vi "3G-PHY-Layer-Complete-System.vi"() -> ()   [LabVIEW 2017]
uses:
  <vilib>/addons/Modulation/Digital/Channel Coding/MT Convolutional Encoder (Rate).vi
  <vilib>/addons/Modulation/Analog/support/mod_Set Error Source.vi
  <vilib>/addons/Modulation/Digital/Support/Common/Validators/mod_Validate Bit Stream.vi
  <vilib>/addons/Modulation/Digital/Channel Coding/Convolutional codes/mod_Convolutional encoder.vi
  <vilib>/addons/Modulation/Digital/Support/Common/Validators/mod_AWGN Validate.vi
  <vilib>/addons/Modulation/Digital/Impairments/subVIs/mod_createSeeds.vi
  <vilib>/addons/Modulation/Digital/Channel Coding/Convolutional codes/subVIs/mod_Generate encoder tap connections.vi
  <vilib>/addons/Modulation/Digital/Channel Coding/Convolutional codes/subVIs/mod_Perform convolutional encoding.vi
  <vilib>/addons/Modulation/Digital/Channel Coding/Block codes/subVIs/mod_Buffer block code info (I8).vi
  <vilib>/addons/Modulation/Digital/Channel Coding/Convolutional codes/subVIs/mod_Generate valid reset (convolutional, I8).vi
  <vilib>/addons/Modulation/Digital/Support/Common/Validators/mod_Validate Samples Per Symbol.vi
  <vilib>/addons/Modulation/Analog/support/Validators/mod_Validate Complex Waveform.vi
  <vilib>/addons/Modulation/Analog/support/Validators/mod_WFErrorHandler.vi
  <vilib>/addons/Modulation/Digital/General/MT Generate Bits (Fibonacci, PN Order).vi
  <vilib>/addons/Modulation/Digital/Support/Common/Validators/mod_Generate Filter Coefficients Validate.vi
  <vilib>/addons/Modulation/Digital/General/subVIs/mod_Generate Filter Coefficients.vi
  <vilib>/addons/Modulation/Digital/General/MT Generate PSK System Parameters(M).vi
  <vilib>/addons/Modulation/Digital/Channel Coding/Convolutional codes/subVIs/mod_Select known generator matrix.vi
  <vilib>/addons/Modulation/Digital/Support/Common/Validators/mod_Validate Convolutional Encoder prms.vi
  <vilib>/addons/Modulation/Digital/General/MT Generate PSK Synchronization Parameters (bit array).vi
  <vilib>/addons/Modulation/Digital/General/subVIs/mod_Generate Bits PN Sequence.vi
  <vilib>/Analysis/1siggen.llb/Gaussian White Noise (obs 90).vi
  <vilib>/addons/Modulation/Digital/Channel Coding/MT Convolutional Decoder (Viterbi Hard Decision, Rate).vi
  <vilib>/addons/Modulation/Digital/Demodulation/MT Calculate BER After Trigger (Fibonacci PN Sequence).vi
  <vilib>/addons/Modulation/niDMT.lvlib
panel:
  out "accumulated BER":dbl format="%.4f"
  out "BER":dbl format="%.4f"
  out "trigger found index (bits)":u32
  out "Decoding":i8[](graph)
  out "Demodulation":i8[](graph)
  out "Despreading":i8[](graph)
  out "trigger found?":bool
  in  "Eb/N0 (10 dB)":dbl=10.0 format="%.2f"
  out "Constellation Graph 2":T1(graph)
  out "Modulation":cluster{"t0":dbl, "dt":dbl, "Y":dbl[]}(graph)
  out "Spreading":i8[](graph)
  out "Encoding":i8[](graph)
  out "Constellation Graph":T1(graph)
  in  "stop":bool
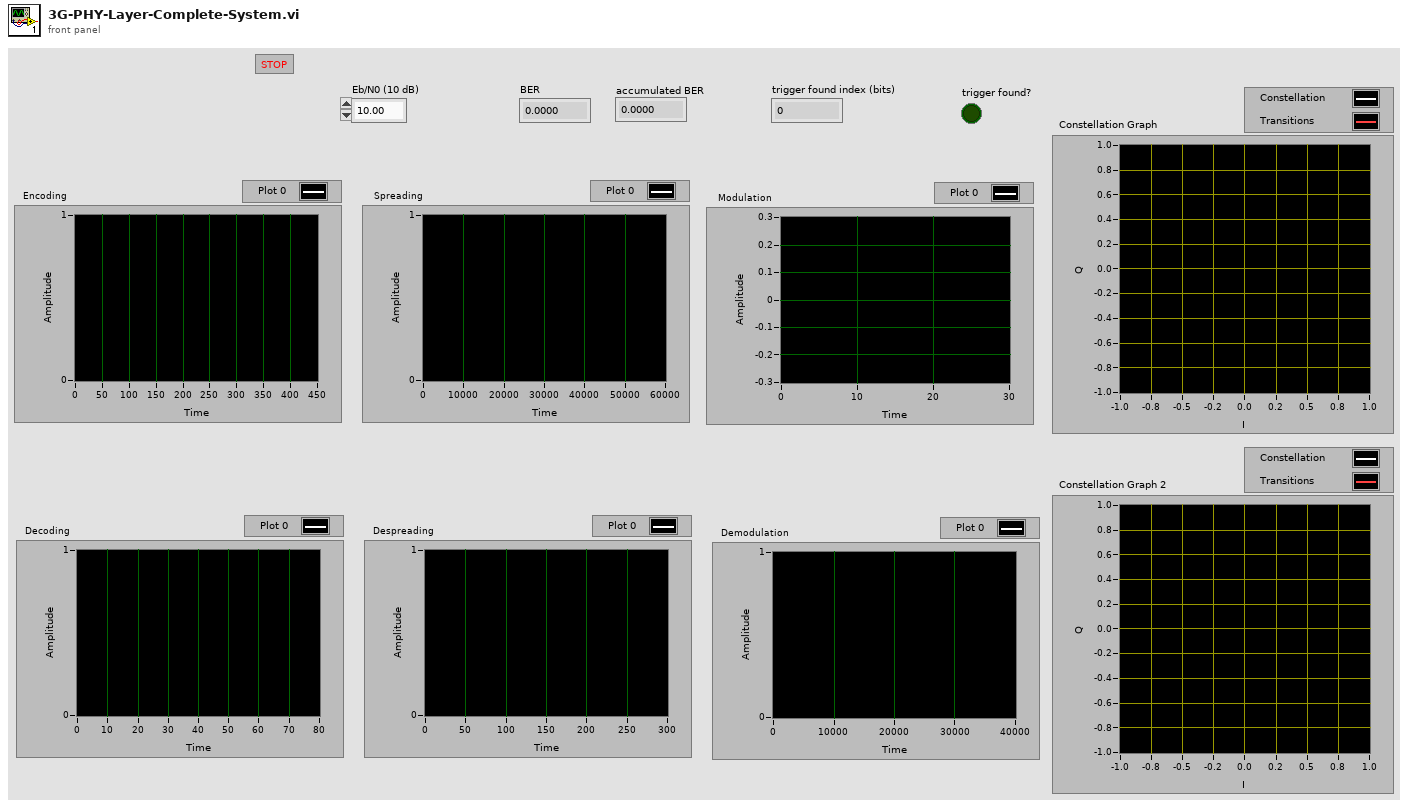
[diagram p1: front panel]
types:
  T1 = cluster{"Decimated Array":dbl[], "Decimated Array":dbl[]}[]
  T2 = enum16{"none", "Raised Cosine", "Root Raised Cos", "Gaussian"}
  T3 = enum16{"FSK", "PSK", "QAM", "MSK", "PAM", "ASK", "CPM"}
  T4 = cluster{"samples per symbol (16)":i32, "symbol map":cdb[], "differential PSK":enum16{"disable", "enable"}, "PSK type":u16}
  T5 = cluster{"expected sync location (symbols)":i32, "sync sequence":cdb[], "sync location uncertainty (symbols)":i32, "sync indent (symbols)":i32}
  T6 = typedef "niAMT.lvlib/Complex Data Waveform.ctl" = cluster{"t0":dbl, "dt":dbl, "Y":cdb[]}
  T7 = cluster{"constellation":dbl[], "oversampled data":dbl[]}[]
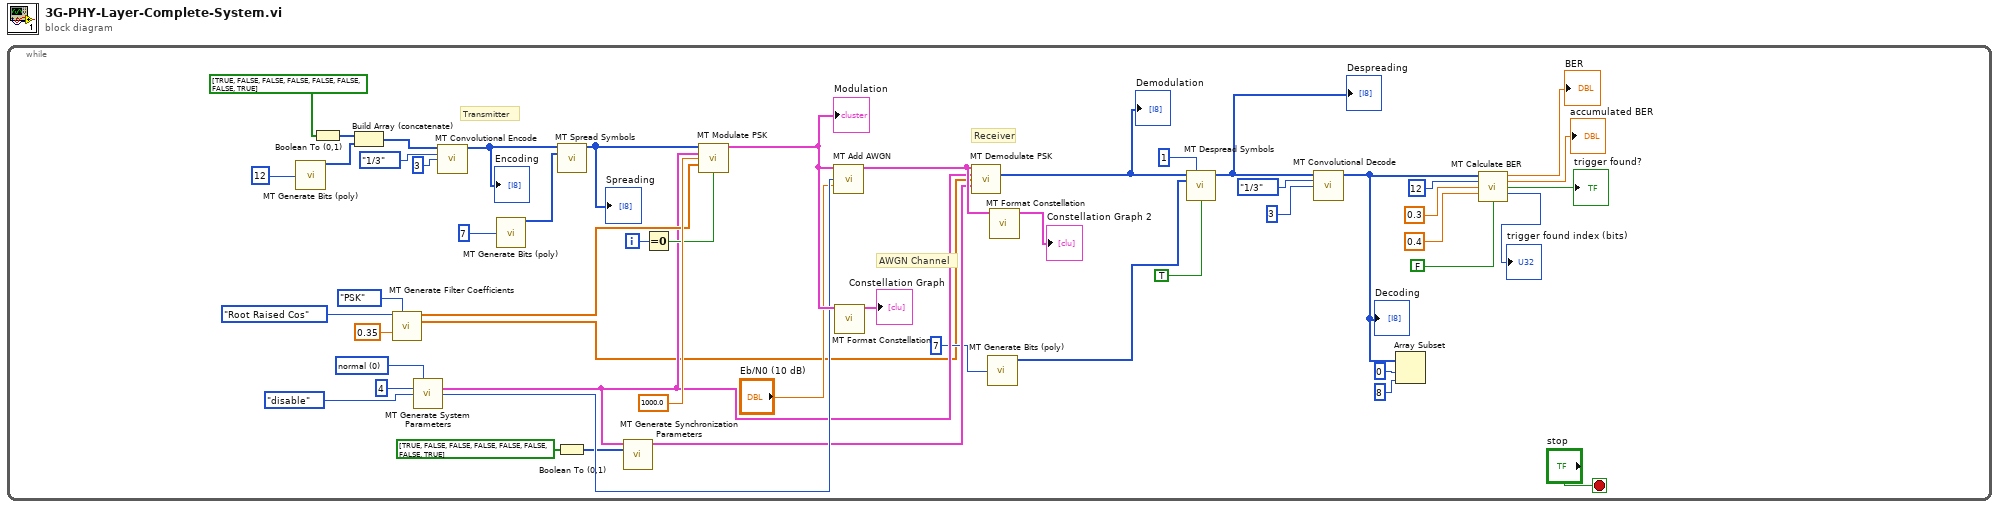
[diagram p0: block diagram]
diagram:
  n1 = while {
    i -> [w37]
    stop <- "stop" stop-if-true
    w49 = u16 0 items=["normal", "shifted", "offset"] ("PSK type")
    # "Receiver"
    # "AWGN Channel"
    # "Transmitter"
    n2 = call-poly <vilib>:"MT Generate Bits (poly).vi"("PN sequence order"=12) -> ("output bit stream"=w9:i8[])  [unwired: 12 in, 2 out]
    n3 = Boolean To (0,1)(Boolean=bool[] [TRUE, FALSE, FALSE, FALSE, FALSE, FALSE, FALSE, TRUE]) -> (0, 1=w39:i16[])
    n4 = Build Array (concatenate) "Build Array"(w39, w9) -> (w34:i16[])
    n5 = call <vilib>:"MT Generate Filter Coefficients.vi"("pulse shaping filter (none)"=T2."Root Raised Cos", "modulation type"=T3."PSK", "filter parameter"=0.35) -> ("pulse shaping filter coefficients"=w27:dbl[], "matched filter coefficients"=w3:dbl[])  [unwired: 10 in, 1 out]
    n6 = call-poly <vilib>:"MT Generate System Parameters.vi"("PSK type"=w49, "M-PSK (4)"=4, "differential PSK"=enum16{"disable", "enable"}."disable") -> ("PSK system parameters"=w26:T4, "bits per symbol"=w29:i32)  [unwired: 10 in, 1 out]
    n7 = call-poly <vilib>:"MT Convolutional Encode.vi"("input bit stream"=w34, "rate (k/n)"=enum16{"1/2", "1/3", "1/4", "2/3", "3/4"}."1/3", "constraint length (K)"=3) -> ("output bit stream"=w32:i8[])  [unwired: 10 in, 2 out]
    "Encoding" <- w32
    n8 = call-poly <vilib>:"MT Generate Bits (poly).vi"("PN sequence order"=7) -> ("output bit stream"=w43:i8[])  [unwired: 12 in, 2 out]
    n9 = Boolean To (0,1)(Boolean=bool[] [TRUE, FALSE, FALSE, FALSE, FALSE, FALSE, FALSE, TRUE]) -> (0, 1=w23:i16[])
    n10 = call <vilib>:"MT Spread Symbols.vi"("input bit stream"=w32, "spreading code"=w43) -> ("output chip stream"=w33:i8[])  [unwired: 12 in, 1 out]
    "Spreading" <- w33
    n11 = call-poly <vilib>:"MT Generate Synchronization Parameters.vi"("PSK system parameters"=w26, "sync bits"=w23) -> ("PSK synchronization parameters"=w25:T5)  [unwired: 12 in, 1 out]
    n12 = Equal To 0?(x=w37) -> (x = 0?=w36:bool)
    n13 = call <vilib>:"MT Modulate PSK.vi"("input bit stream"=w33, "PSK system parameters"=w26, "symbol rate (Hz)"=1000.0, "pulse shaping filter coefficients"=w27, "reset? (T)"=w36) -> ("output complex waveform"=w31:T6)  [unwired: 8 in, 2 out]
    "Modulation" <- w31
    n14 = call <vilib>:"MT Add AWGN.vi"("input complex waveform"=w31, "bits per symbol (1)"=w29, "Eb/N0 (10 dB)"="Eb/N0 (10 dB)") -> ("output complex waveform"=w28:T6)  [unwired: 10 in, 2 out]
    n15 = call <vilib>:"MT Format Constellation.vi"("waveform"=w31) -> ("constellation graph"=→"Constellation Graph":T7)  [unwired: 13 in, 1 out]
    n16 = call <vilib>:"MT Demodulate PSK.vi"("input complex waveform"=w28, "PSK system parameters"=w26, "matched filter coefficients"=w3, "synchronization parameters"=w25) -> ("output bit stream"=w10:i8[])  [unwired: 7 in, 4 out]
    "Demodulation" <- w10
    n17 = call-poly <vilib>:"MT Generate Bits (poly).vi"("PN sequence order"=7) -> ("output bit stream"=w21:i8[])  [unwired: 12 in, 2 out]
    n18 = call <vilib>:"MT Format Constellation.vi"("waveform"=w28) -> ("constellation graph"=→"Constellation Graph 2":T7)  [unwired: 13 in, 1 out]
    n19 = call <vilib>:"MT Despread Symbols.vi"("input chip stream"=w10, "sync search depth (bits)"=1, "spreading code"=w21, "reset? (T)"=TRUE) -> ("output bit stream"=w11:i8[])  [unwired: 8 in, 3 out]
    "Despreading" <- w11
    n20 = call-poly <vilib>:"MT Convolutional Decode.vi"("input bit stream"=w11, "rate (k/n)"=enum16{"1/2", "1/3", "1/4", "2/3", "3/4"}."1/3", "constraint length (K)"=3) -> ("output bit stream"=w5:i8[])  [unwired: 10 in, 2 out]
    "Decoding" <- w5
    n21 = Array Subset(array=w5, index=0, length=8) -> ()  [unwired: 1 out]
    n22 = call-poly <vilib>:"MT Calculate BER.vi"("input bit stream"=w5, "PN sequence order (9)"=12, "BER trigger threshold (0.1)"=0.3, "confidence (0.95)"=0.4, "reset? (T)"=FALSE) -> ("BER"=→"BER":dbl, "accumulated BER"=→"accumulated BER":dbl, "trigger found?"=→"trigger found?":bool, "trigger found index (bits)"=→"trigger found index (bits)":u32)  [unwired: 6 in, 1 out]
  }
